vi "New Project.vi"(9 "DBSet":T1={"Server"="172.20.23.107", "DB"="HTPSDB", "PSW"="data'songyy", "User"="sa"}, 10 "UserID":string="L043460", 11 "厂区":string="清溪") -> ()   [LabVIEW 2011] (continued)
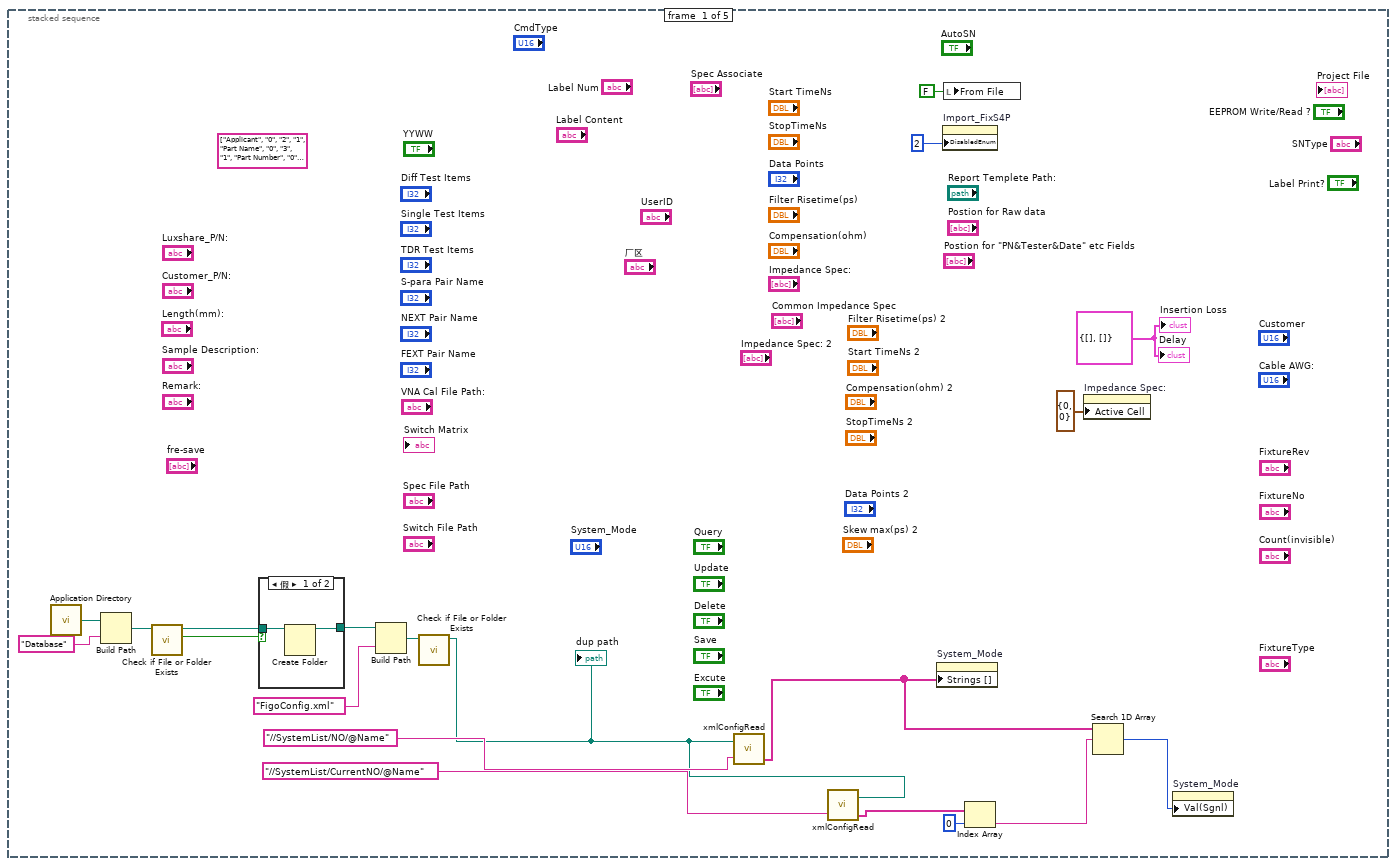
[diagram p3: hidden frame]
                            n930 = Build Array(w1122, w1135, w1134, w1133, w1132, w1131, w1130, w1129, w1128, w1127, w1110, w1112, w1123, w1126, w1138, w1125, w1124, w1119, w1107, w1108, w1109, w1105) -> (w1114:string[])
                            n931 = local write "Project File"(w1114) -> ()
                          }
                        }
                      }
                      frame #4 {
                        n932 = local read "save?"() -> (w1140:bool)
                        n933 = case shown="真" w1140 {
                          tunnel: w1139 -> [_ w1142]
                          frame False {
                            n934 = One Button Dialog(message="保存信息不完整" ("消息")) -> ()  [unwired: 1 in, 1 out]
                          }
                          frame True {
                            n935 = local read "Luxshare_P/N:"() -> (w1145:string)
                            n936 = local read "Project File"() -> (w1144:string[])
                            n937 = local read "Local"() -> (w1143:bool)
                            n938 = case shown="真" w1143 {
                              tunnel: w1144 -> [w1150 w1162]
                              tunnel: w1145 -> [_ w1170]
                              tunnel: w1142 -> [w1146 _]
                              frame False {
                                (unwired) string[] ["LuxsharePN", "CustomerPN", "Customer", "Prjinf", "SampleDes", "AWG", "Length", "Spec", "SwitchMatrix", "EEPROMTF", "FixtureNo", "LabelTF", "LabelNum", "LabelC", "Remark", "AutoSN", "FrePoints"] ("列名")
                                # "保存至数据库"
                                n939 = call "sql-writeinfo_vproject.vi"("操作模式"=enum16{"写入数据", "更改数据"}."写入数据", "列名"=string[] ["LuxsharePN", "CustomerPN", "Customer", "Prjinf", "SampleDes", "AWG", "Length", "Spec", "SwitchMatrix", "EEPROMTF", "FixtureNo", "LabelTF", "LabelNum", "LabelC", "Remark", "AutoSN", "FrePoints", "Switch_File_Path", "Spec_File_Path", "Spec_Points", "HardWare_Mode", "Factory", "LastLog"], "DBSet"=w1146, "值"=w1150) -> ("简单报错"=w1148:string, "status"=w1149:bool)  [unwired: 14 in]
                                n940 = case shown="假" w1149 {
                                tunnel: w1148 -> [_ w1161]
                                frame False {
                                # "清空操作"
                                n941 = control-ref of="Spec Associate"() -> (w1152:refnum<vi>)
                                n942 = control-ref of="Report Templete Path:"() -> (w1155:refnum<vi>)
                                n943 = control-ref of="Data Points"() -> (w1154:refnum<vi>)
                                n944 = local read "bool"() -> (w1153:refnum<vi>[])
                                n945 = One Button Dialog(message="Save Finished!" ("消息")) -> ()  [unwired: 1 in, 1 out]
                                n946 = local read "number"() -> (w1156:refnum<vi>[])
                                n947 = local read "string"() -> (w1159:refnum<vi>[])
                                n948 = local read "chart"() -> (w1157:refnum<vi>[])
                                n949 = local read "list"() -> (w1158:refnum<vi>[])
                                n950 = call "_wmg_initAllCtrls.vi"("chart"=w1157, "number"=w1156, "list"=w1158, "string"=w1159, "bool"=w1153, "Spec _Data"=w1152, "Data Points"=w1154, "Report Templete Path:"=w1155) -> ()
                                }
                                frame True {
                                n951 = One Button Dialog(message=w1161) -> ()  [unwired: 1 in, 1 out]
                                }
                                }
                              }
                              frame True {
                                n952 = call <vilib>:"Application Directory.vi"() -> ("Application Directory"=w1169:path)
                                n953 = Concatenate Strings("Database\\" ("字符串"), w1170, ".hpj" ("字符串")) -> (w1168:string)
                                n954 = Build Path(base path=w1169, name or relative path=w1168) -> (appended path=w1165:path)
                                n955 = call <vilib>:"Check if File or Folder Exists.vi"("path"=w1165) -> ("file or folder exists?"=w1164:bool, "dup path"=w1163:path)  [unwired: 8 in, 1 out]
                                n956 = case shown="真" w1164 {
                                tunnel: w1163 -> [w1174 w1184]
                                tunnel: w1162 -> [w1173 w1183]
                                frame False {
                                # "清空操作"
                                n957 = control-ref of="Spec Associate"() -> (w1171:refnum<vi>)
                                n958 = One Button Dialog(message="Local file save Finished!" ("消息")) -> ()  [unwired: 1 in, 1 out]
                                n959 = control-ref of="Report Templete Path:"() -> (w1180:refnum<vi>)
                                n960 = control-ref of="Data Points"() -> (w1181:refnum<vi>)
                                n961 = local read "bool"() -> (w1172:refnum<vi>[])
                                n962 = Write to Binary File(file (use dialog)=w1174, data=w1173, 9:T8."big-endian, network order" ("字节顺序(0:big-endian, network order)")) -> ()  [unwired: 3 in, 3 out]
                                n963 = local read "number"() -> (w1179:refnum<vi>[])
                                n964 = local read "string"() -> (w1176:refnum<vi>[])
                                n965 = local read "chart"() -> (w1178:refnum<vi>[])
                                n966 = local read "list"() -> (w1177:refnum<vi>[])
                                n967 = call "_wmg_initAllCtrls.vi"("chart"=w1178, "number"=w1179, "list"=w1177, "string"=w1176, "bool"=w1172, "Spec _Data"=w1171, "Data Points"=w1181, "Report Templete Path:"=w1180) -> ()
                                }
                                frame True {
                                n968 = Two Button Dialog(message="该PN的文件已经存在\n是否覆盖？", 1:"取消" ("F按钮名称（“取消”）"), 2:"覆盖" ("T按钮名称（“确定”）")) -> (T button?=w1185:bool)
                                n969 = case shown="真" w1185 {
                                tunnel: w1184 -> [_ w1190]
                                tunnel: w1183 -> [_ w1189]
                                frame False {
                                }
                                frame True {
                                n970 = stacked-sequence {
                                tunnel: w1190 -> [w1193 _]
                                tunnel: w1189 -> [w1191 _]
                                frame #0 {
                                n971 = One Button Dialog(message="Coved successfully!" ("消息")) -> ()  [unwired: 1 in, 1 out]
                                n972 = Write to Binary File(file (use dialog)=w1193, data=w1191, 9:T8."big-endian, network order" ("字节顺序(0:big-endian, network order)")) -> ()  [unwired: 3 in, 3 out]
                                }
                                frame #1 {
                                # "清空操作"
                                n973 = control-ref of="Report Templete Path:"() -> (w1200:refnum<vi>)
                                n974 = control-ref of="Data Points"() -> (w1201:refnum<vi>)
                                n975 = control-ref of="Spec Associate"() -> (w1195:refnum<vi>)
                                n976 = local read "number"() -> (w1199:refnum<vi>[])
                                n977 = local read "string"() -> (w1196:refnum<vi>[])
                                n978 = local read "chart"() -> (w1198:refnum<vi>[])
                                n979 = local read "list"() -> (w1197:refnum<vi>[])
                                n980 = call "_wmg_initAllCtrls.vi"("chart"=w1198, "number"=w1199, "list"=w1197, "string"=w1196, "Spec _Data"=w1195, "Data Points"=w1201, "Report Templete Path:"=w1200) -> ()  [unwired: 1 in]
                                }
                                }
                                }
                                }
                                }
                                }
                              }
                            }
                          }
                        }
                      }
                      frame #5 {
                        n981 = property on="Update" class="Bool (严格)"("DisabledEnum"=T5."Disabled and Grayed Out" ("禁用")) -> ()  [unwired: 2 in, 2 out]
                        n982 = property on="Delete" class="Bool (严格)"("DisabledEnum"=T5."Disabled and Grayed Out" ("禁用")) -> ()  [unwired: 2 in, 2 out]
                        n983 = property on="Luxshare_P/N:" class="Str"("DisabledEnum"=T5."Disabled and Grayed Out" ("禁用")) -> ()  [unwired: 2 in, 2 out]
                        n984 = local write "Delete"(FALSE ("Query")) -> ()
                        n985 = local write "Save"(FALSE ("Query")) -> ()
                        n986 = local write "Query"(FALSE ("Query")) -> ()
                        n987 = local write "Update"(FALSE ("Query")) -> ()
                      }
                    }
                  }
                  frame #2 {
                    w1210 = u16 0 items=["", "Common", "H3C psw 10G", "H3C psw 28G"] ("CmdType")
                    # "清空数组"
                    n988 = control-ref of="Spec Associate"() -> (w1209:refnum<vi>)
                    n989 = control-ref of="Report Templete Path:"() -> (w1213:refnum<vi>)
                    n990 = control-ref of="Data Points"() -> (w1212:refnum<vi>)
                    n991 = local write "CmdType"(w1210) -> ()
                    n992 = local read "bool"() -> (w1211:refnum<vi>[])
                    n993 = local read "number"() -> (w1214:refnum<vi>[])
                    n994 = local read "string"() -> (w1217:refnum<vi>[])
                    n995 = local read "chart"() -> (w1215:refnum<vi>[])
                    n996 = local read "list"() -> (w1216:refnum<vi>[])
                    n997 = call "_wmg_initAllCtrls.vi"("chart"=w1215, "number"=w1214, "list"=w1216, "string"=w1217, "bool"=w1211, "Spec _Data"=w1209, "Data Points"=w1212, "Report Templete Path:"=w1213) -> ()
                    n998 = property on="Update" class="Bool (严格)"("DisabledEnum"=T5."Disabled and Grayed Out" ("禁用")) -> ()  [unwired: 2 in, 2 out]
                    n999 = property on="Delete" class="Bool (严格)"("DisabledEnum"=T5."Disabled and Grayed Out" ("禁用")) -> ()  [unwired: 2 in, 2 out]
                    n1000 = property on="Luxshare_P/N:" class="Str"("DisabledEnum"=T5."Disabled and Grayed Out" ("禁用")) -> ()  [unwired: 2 in, 2 out]
                    n1001 = local write "Delete"(FALSE ("Query")) -> ()
                    n1002 = local write "Save"(FALSE ("Query")) -> ()
                    n1003 = local write "Query"(FALSE ("Query")) -> ()
                    n1004 = local write "Update"(FALSE ("Query")) -> ()
                  }
                }
              }
              frame 10 {
                n1005 = stacked-sequence {
                  tunnel: w1225 -> [w1226 _]
                  frame #0 {
                    n1006 = local read "Local"() -> (w1227:bool)
                    n1007 = case shown="假" w1227 {
                      tunnel: w1226 -> [w1228 _]
                      frame False {
                        n1008 = local read "Luxshare_P/N:"() -> (w1237:string)
                        n1009 = property on="System_Mode" class="Ring (严格)"() -> ("RingText.Text"=w1233:string)  [unwired: 2 in, 2 out]
                        n1010 = local read "厂区"() -> (w1229:string)
                        n1011 = call "_wmg_HardModetoHardModewhereConnect.vi"("Input"=w1233, "Factory"=w1229) -> ("Output"=w1231:string)
                        n1012 = call "_wmg_PNtoPNwhereConnect.vi"("Input"=w1237) -> ("Output"=w1232:string)
                        n1013 = Concatenate Strings(w1232, w1231) -> (w1230:string)
                        n1014 = call "sql-delete.vi"("操作模式"=T9."删除数据", "DBSet"=w1228, "限定条件"=w1230) -> ("错误类型"=w1234:string, "status"=w1235:bool)  [unwired: 15 in]
                        n1015 = case shown="假" w1235 {
                          tunnel: ["数据删除成功！" ("消息") w1240] -> w1236
                          tunnel: w1234 -> [_ w1240]
                          frame False {
                          }
                          frame True {
                          }
                        }
                        n1016 = One Button Dialog(message=w1236) -> ()  [unwired: 1 in, 1 out]
                      }
                      frame True {
                        n1017 = local read "Luxshare_P/N:"() -> (w1246:string)
                        n1018 = call <vilib>:"Application Directory.vi"() -> ("Application Directory"=w1250:path)
                        n1019 = Concatenate Strings("Database\\" ("字符串"), w1246, ".hpj" ("字符串")) -> (w1249:string)
                        n1020 = Build Path(base path=w1250, name or relative path=w1249) -> (appended path=w1245:path)
                        n1021 = Delete(path (use dialog)=w1245) -> (error out=w1241:errorcluster)  [unwired: 4 in, 2 out]
                        n1022 = Unbundle(w1241) -> ("status"=w1244:bool, "source"=w1242:string)  [unwired: 1 out]
                        n1023 = case shown="假" w1244 {
                          tunnel: ["文件删除成功！" ("消息") w1252] -> w1243
                          tunnel: w1242 -> [_ w1252]
                          frame False {
                          }
                          frame True {
                          }
                        }
                        n1024 = One Button Dialog(message=w1243) -> ()  [unwired: 1 in, 1 out]
                      }
                    }
                  }
                  frame #1 {
                    w1254 = u16 0 items=["", "Common", "H3C psw 10G", "H3C psw 28G"] ("CmdType")
                    # "清空数组"
                    n1025 = control-ref of="Spec Associate"() -> (w1253:refnum<vi>)
                    n1026 = control-ref of="Report Templete Path:"() -> (w1264:refnum<vi>)
                    n1027 = control-ref of="Data Points"() -> (w1263:refnum<vi>)
                    n1028 = local write "CmdType"(w1254) -> ()
                    n1029 = local read "bool"() -> (w1255:refnum<vi>[])
                    n1030 = local read "number"() -> (w1265:refnum<vi>[])
                    n1031 = local read "string"() -> (w1268:refnum<vi>[])
                    n1032 = local read "chart"() -> (w1266:refnum<vi>[])
                    n1033 = local read "list"() -> (w1267:refnum<vi>[])
                    n1034 = call "_wmg_initAllCtrls.vi"("chart"=w1266, "number"=w1265, "list"=w1267, "string"=w1268, "bool"=w1255, "Spec _Data"=w1253, "Data Points"=w1263, "Report Templete Path:"=w1264) -> ()
                    n1035 = local write "Delete"(FALSE ("Query")) -> ()
                    n1036 = property on="Update" class="Bool (严格)"("DisabledEnum"=T5."Disabled and Grayed Out" ("禁用")) -> ()  [unwired: 2 in, 2 out]
                    n1037 = property on="Delete" class="Bool (严格)"("DisabledEnum"=T5."Disabled and Grayed Out" ("禁用")) -> ()  [unwired: 2 in, 2 out]
                    n1038 = property on="Luxshare_P/N:" class="Str"("DisabledEnum"=T5."Disabled and Grayed Out" ("禁用")) -> ()  [unwired: 2 in, 2 out]
                    n1039 = local write "Save"(FALSE ("Query")) -> ()
                    n1040 = local write "Query"(FALSE ("Query")) -> ()
                    n1041 = local write "Update"(FALSE ("Query")) -> ()
                  }
                }
              }
              frame 1 {
                n1042 = stacked-sequence {
                  tunnel: w1269 -> [_ _ _ _ w1451 _]
                  frame #0 {
                    w1296 = "@"
                    w1297 = "\r\n"
                    w1307 = "%s" ("格式字符串")
                    n1043 = local read "Impedance Spec:"() -> (w1309:string[][])
                    n1044 = local read "2X Thru String"() -> (w1293:string)
                    n1045 = property on="Delay(ns)" class="DigNum (严格)"() -> ("NumText.Text"=w1291:string)  [unwired: 2 in, 2 out]
                    n1046 = property on="Skew max(ps)" class="DigNum (严格)"() -> ("NumText.Text"=w1292:string)  [unwired: 2 in, 2 out]
                    n1047 = Boolean To (0,1)(Boolean="Impedance Filter") -> (0, 1=w1312:i16)
                    n1048 = property on="Filter Risetime(ps)" class="DigNum (严格)"() -> ("NumText.Text"=w1287:string)  [unwired: 2 in, 2 out]
                    n1049 = property on="Start TimeNs" class="DigNum (严格)"() -> ("NumText.Text"=w1290:string)  [unwired: 2 in, 2 out]
                    n1050 = property on="StopTimeNs" class="DigNum (严格)"() -> ("NumText.Text"=w1289:string)  [unwired: 2 in, 2 out]
                    n1051 = property on="Data Points" class="DigNum (严格)"() -> ("NumText.Text"=w1288:string)  [unwired: 2 in, 2 out]
                    n1052 = property on="Compensation(ohm)" class="DigNum (严格)"() -> ("NumText.Text"=w1286:string)  [unwired: 2 in, 2 out]
                    n1053 = Number To Decimal String(number=w1312) -> (decimal integer string=w1310:string)  [unwired: 1 in]
                    n1054 = call "impedance spec.vi"("Impedance Spec:"=w1309) -> ("Impedance spec string"=w1308:string)  [unwired: 10 in]
                    n1055 = call <vilib>:"Trim Whitespace.vi"("string"=w1293) -> ("trimmed string"=w1285:string)  [unwired: 1 in]
                    n1056 = Build Array(w1290, w1289, w1288, w1287, w1286, w1310, w1308, w1291, w1292, w1285) -> (→"TDR Setting":string[])
                    n1057 = local read "Impedance Spec: 2"() -> (w1275:string[][])
                    n1058 = local read "Report Templete Path:"() -> (w1294:path)
                    n1059 = local read "2X Thru String"() -> (w1282:string)
                    n1060 = property on="Delay(ns)" class="DigNum (严格)"() -> ("NumText.Text"=w1273:string)  [unwired: 2 in, 2 out]
                    n1061 = property on="Skew max(ps) 2" class="DigNum (严格)"() -> ("NumText.Text"=w1272:string)  [unwired: 2 in, 2 out]
                    n1062 = property on="Postion for Raw data" class="Tbl (严格)"() -> ("Value"=w1306:string[][])  [unwired: 2 in, 2 out]
                    n1063 = property on="Start TimeNs 2" class="DigNum (严格)"() -> ("NumText.Text"=w1281:string)  [unwired: 2 in, 2 out]
                    n1064 = property on="StopTimeNs 2" class="DigNum (严格)"() -> ("NumText.Text"=w1280:string)  [unwired: 2 in, 2 out]
                    n1065 = property on="Data Points 2" class="DigNum (严格)"() -> ("NumText.Text"=w1279:string)  [unwired: 2 in, 2 out]
                    n1066 = property on="Postion for \"PN&Tester&Date\" etc Fields" class="Tbl (严格)"() -> ("Value"=w1305:string[][])  [unwired: 2 in, 2 out]
                    n1067 = property on="Filter Risetime(ps) 2" class="DigNum (严格)"() -> ("NumText.Text"=w1278:string)  [unwired: 2 in, 2 out]
                    n1068 = property on="Compensation(ohm) 2" class="DigNum (严格)"() -> ("NumText.Text"=w1277:string)  [unwired: 2 in, 2 out]
                    n1069 = Boolean To (0,1)(Boolean="Impedance Filter 2") -> (0, 1=w1283:i16)
                    n1070 = Array To Spreadsheet String(array=w1306, 3:w1307) -> (spreadsheet string=w1302:string)  [unwired: 1 in]
                    n1071 = Array To Spreadsheet String(array=w1305, 3:w1307) -> (spreadsheet string=w1300:string)  [unwired: 1 in]
                    n1072 = Number To Decimal String(number=w1283) -> (decimal integer string=w1276:string)  [unwired: 1 in]
                    n1073 = call "impedance spec.vi"("Impedance Spec:"=w1275) -> ("Impedance spec string"=w1274:string)  [unwired: 10 in]
                    n1074 = call <vilib>:"Trim Whitespace.vi"("string"=w1282) -> ("trimmed string"=w1271:string)  [unwired: 1 in]
                    n1075 = Path To String(path=w1294) -> (string=w1295:string)
                    n1076 = Search and Replace String(replace all?=TRUE ("替换全部？(F)"), input string=w1302, search string=w1297, replace string=w1296) -> (result string=w1299:string)  [unwired: 4 in, 3 out]
                    n1077 = Search and Replace String(replace all?=TRUE ("替换全部？(F)"), input string=w1300, search string=w1297, replace string=w1296) -> (result string=w1298:string)  [unwired: 4 in, 3 out]
                    n1078 = Build Array(w1281, w1280, w1279, w1278, w1277, w1276, w1274, w1273, w1272, w1271) -> (→"TDR Setting2":string[])
                    n1079 = Build Array(w1295, w1299, w1298) -> (→"Report Config":string[])
                  }
                  frame #1 {
                    n1080 = property on="S-para Pair Name" class="LstBox (严格)"() -> ("Item Names"=w1349:string[], "Item Symbols"=w1348:i32[])  [unwired: 2 in, 2 out]
                    n1081 = property on="NEXT Pair Name" class="LstBox (严格)"() -> ("Item Names"=w1347:string[], "Item Symbols"=w1346:i32[])  [unwired: 2 in, 2 out]
                    n1082 = local read "Common Impedance Spec"() -> (w1317:string[][])
                    n1083 = property on="FEXT Pair Name" class="LstBox (严格)"() -> ("Item Names"=w1345:string[], "Item Symbols"=w1344:i32[])  [unwired: 2 in, 2 out]
                    n1084 = property on="Single Test Items" class="LstBox (严格)"() -> ("Item Names"=w1351:string[], "Item Symbols"=w1350:i32[])  [unwired: 2 in, 2 out]
                    n1085 = property on="Diff Test Items" class="LstBox (严格)"() -> ("Item Names"=w1353:string[], "Item Symbols"=w1352:i32[])  [unwired: 2 in, 2 out]
                    n1086 = property on="TDR Test Items" class="LstBox (严格)"() -> ("Item Names"=w1329:string[], "Item Symbols"=w1328:i32[])  [unwired: 2 in, 2 out]
                    n1087 = call "Selected items.vi"("Item Syms"=w1348, "Item name"=w1349) -> ("Selected tem"=w1343:string[])  [unwired: 7 in, 2 out]
                    n1088 = call "Selected items.vi"("Item Syms"=w1346, "Item name"=w1347) -> ("Selected tem"=w1342:string[])  [unwired: 7 in, 2 out]
                    n1089 = call "Selected items.vi"("Item Syms"=w1344, "Item name"=w1345) -> ("Selected tem"=w1341:string[])  [unwired: 7 in, 2 out]
                    n1090 = call "Selected items.vi"("Item Syms"=w1352, "Item name"=w1353) -> ("Selected tem"=w1340:string[])  [unwired: 7 in, 2 out]
                    n1091 = call "Selected items.vi"("Item Syms"=w1350, "Item name"=w1351) -> ("Selected tem"=w1339:string[])  [unwired: 7 in, 2 out]
                    n1092 = call "Selected items.vi"("Item Syms"=w1328, "Item name"=w1329) -> ("Selected tem"=w1327:string[])  [unwired: 7 in, 2 out]
                    n1093 = call "impedance spec.vi"("Impedance Spec:"=w1317) -> ("Impedance spec string"=w1316:string)  [unwired: 10 in]
                    n1094 = local read "VNA Cal File Path:"() -> (w1324:string)
                    n1095 = Build Array(w1316) -> (w1315:string[])
                    n1096 = local read "Report Config"() -> (w1325:string[])
                    n1097 = local read "Cancel Dem2X?"() -> (w1322:bool)
                    n1098 = local read "TDR Setting2"() -> (w1323:string[])
                    n1099 = local read "TDR Setting"() -> (w1326:string[])
                    n1100 = Build Array(w1324) -> (w1338:string[])
                    n1101 = Number To Decimal String(number="ILD Spec") -> (decimal integer string=w1331:string)  [unwired: 1 in]
                    n1102 = Build Array(w1331) -> (w1330:string[])
                    n1103 = Select(t="TRUE", s=w1322, f="FALSE") -> (s? t:f=w1319:string)
                    n1104 = Build Array(w1319) -> (w1318:string[])
                    n1105 = Build Array(w1343, w1342, w1341, w1340, w1339, w1327, string[] ["占位符"], w1338, w1325, w1330, w1326, w1323, w1318, w1315) -> (w1337:string[][])
                    n1106 = Transpose 2D Array(2D array=w1337) -> (transposed array=w1336:string[][])
                    n1107 = Array To Spreadsheet String(delimiter (Tab)="#" ("分隔符(Tab)"), array=w1336, 3:"%s" ("格式字符串")) -> (spreadsheet string=→"Project Information":string)
                  }
                  frame #2 {
                    n1108 = local read "VNA Cal File Path:"() -> (w1373:string)
                    n1109 = property on="Diff Test Items" class="LstBox (严格)"() -> ("Item Symbols"=w1370:i32[])  [unwired: 2 in, 2 out]
                    n1110 = property on="Single Test Items" class="LstBox (严格)"() -> ("Item Symbols"=w1369:i32[])  [unwired: 2 in, 2 out]
                    n1111 = property on="TDR Test Items" class="LstBox (严格)"() -> ("Item Symbols"=w1368:i32[])  [unwired: 2 in, 2 out]
                    n1112 = property on="S-para Pair Name" class="LstBox (严格)"() -> ("Item Symbols"=w1367:i32[])  [unwired: 2 in, 2 out]
                    n1113 = property on="NEXT Pair Name" class="LstBox (严格)"() -> ("Item Symbols"=w1366:i32[])  [unwired: 2 in, 2 out]
                    n1114 = property on="FEXT Pair Name" class="LstBox (严格)"() -> ("Item Symbols"=w1362:i32[])  [unwired: 2 in, 2 out]
                    n1115 = local read "Luxshare_P/N:"() -> (w1360:string)
                    n1116 = local read "Length(mm):"() -> (w1374:string)
                    n1117 = String Length(string=w1360) -> (length=w1361:i32)
                    n1118 = Empty String/Path?(string/path=w1373) -> (empty?=w1371:bool)
                    n1119 = Empty String/Path?(string/path=w1374) -> (empty?=w1372:bool)
                    n1120 = Build Array(w1370, w1369, w1368, w1367, w1366, w1362) -> (w1365:i32[][])
                    n1121 = Not(x=w1372) -> (.not. x?=w1364:bool)
                    n1122 = Not(x=w1371) -> (.not. x?=w1363:bool)
                    n1123 = Greater Than 0?(x=w1361) -> (x > 0?=w1359:bool)
                    n1124 = local read "Spec Associate"() -> (w1354:string[][])
                    n1125 = call "_wmg_whetherItemsEmpty.vi"("Input"=w1365) -> ("bool"=w1375:bool)
                    n1126 = Compound Arithmetic op=AND(w1359, w1364, w1363, w1375) -> (→"save?":bool)
                    n1127 = Array To Spreadsheet String(delimiter (Tab)="#" ("分隔符(Tab)"), array=w1354, 3:"%s" ("格式字符串")) -> (spreadsheet string=w1357:string)
                    n1128 = local write "Spec String"(w1357) -> ()
                  }
                  frame #3 {
                    n1129 = local read "Local"() -> (w1376:bool)
                    n1130 = case shown="真" w1376 {
                      frame False {
                        # "16"
                        # "15"
                        # "14"
                        # "13"
                        # "11"
                        # "10"
                        # "9"
                        # "8"
                        # "7"
                        # "6"
                        # "5"
                        # "4"
                        # "3"
                        # "2"
                        # "1"
                        n1131 = local read "Label Print?"() -> (w1388:bool)
                        n1132 = local read "UserID"() -> (w1380:string)
                        n1133 = local read "fre-save"() -> (w1395:string[])
                        n1134 = Format Date/Time String(time format string (%c)="%Y-%m-%d : %H:%M" ("时间格式字符串(%c)")) -> (date/time string=w1377:string)  [unwired: 2 in]
                        n1135 = Boolean To (0,1)(Boolean=w1388) -> (0, 1=w1413:i16)
                        n1136 = local read "EEPROM Write/Read ?"() -> (w1389:bool)
                        n1137 = local read "Sample Description:"() -> (w1409:string)
                        n1138 = local read "Project Information"() -> (w1410:string)
                        n1139 = Array To Spreadsheet String(delimiter (Tab)="," ("分隔符(Tab)"), array=w1395, 3:"" ("格式字符串")) -> (spreadsheet string=w1392:string)
                        n1140 = Number To Decimal String(number=w1413) -> (decimal integer string=w1403:string)  [unwired: 1 in]
                        n1141 = local read "Customer_P/N:"() -> (w1412:string)
                        n1142 = local read "Switch Matrix"() -> (w1405:string)
                        n1143 = local read "Label Content"() -> (w1402:string)
                        n1144 = local read "Length(mm):"() -> (w1407:string)
                        n1145 = local read "Spec String"() -> (w1406:string)
                        n1146 = call <vilib>:"Trim Whitespace.vi"("string"=w1392) -> ("trimmed string"=w1391:string)  [unwired: 1 in]
                        n1147 = Concatenate Strings(w1380, " saved@" ("字符串"), w1377) -> (w1379:string)
                        n1148 = property on="Customer" class="Ring (严格)"() -> ("RingText.Text"=w1411:string)  [unwired: 2 in, 2 out]
                        n1149 = property on="Cable AWG:" class="Ring (严格)"() -> ("RingText.Text"=w1408:string)  [unwired: 2 in, 2 out]
                        n1150 = local read "FixtureNo"() -> (w1400:string)
                        n1151 = local read "Label Num"() -> (w1415:string)
                        n1152 = local read "Remark:"() -> (w1401:string)
                        n1153 = local read "厂区"() -> (w1382:string)
                        n1154 = local read "Switch File Path"() -> (w1387:string)
                        n1155 = Boolean To (0,1)(Boolean=w1389) -> (0, 1=w1414:i16)
                        n1156 = local read "AutoSN"() -> (w1397:bool)
                        n1157 = Number To Decimal String(number=w1414) -> (decimal integer string=w1404:string)  [unwired: 1 in]
                        n1158 = Boolean To (0,1)(Boolean=w1397) -> (0, 1=w1398:i16)
                        n1159 = local read "Spec File Path"() -> (w1386:string)
                        n1160 = Number To Decimal String(number=w1398) -> (decimal integer string=w1396:string)  [unwired: 1 in]
                        n1161 = local read "Luxshare_P/N:"() -> (w1399:string)
                        n1162 = local read "Spec Points"() -> (w1385:dbl)
                        n1163 = property on="System_Mode" class="Ring (严格)"() -> ("RingText.Text"=w1383:string)  [unwired: 2 in, 2 out]
                        n1164 = Number To Decimal String(number=w1385) -> (decimal integer string=w1384:string)  [unwired: 1 in]
                        n1165 = Build Array(w1399, w1412, w1411, w1410, w1409, w1408, w1407, w1406, w1405, w1404, w1400, w1403, w1415, w1402, w1401, w1396, w1391, w1387, w1386, w1384, w1383, w1382, w1379) -> (w1390:string[])
                        n1166 = local write "Project File"(w1390) -> ()
                      }
                      frame True {
                        # "11"
                        # "10"
                        # "9"
                        # "8"
                        # "7"
                        # "6"
                        # "5"
                        # "4"
                        # "3"
                        # "2"
                        # "1"
                        n1167 = local read "Label Print?"() -> (w1421:bool)
                        n1168 = local read "fre-save"() -> (w1429:string[])
                        n1169 = Boolean To (0,1)(Boolean=w1421) -> (0, 1=w1448:i16)
                        n1170 = local read "EEPROM Write/Read ?"() -> (w1423:bool)
                        n1171 = property on="CmdType" class="Ring (严格)"() -> ("RingText.Text"=w1420:string)  [unwired: 2 in, 2 out]
                        n1172 = local read "Sample Description:"() -> (w1444:string)
                        n1173 = local read "Project Information"() -> (w1445:string)
                        n1174 = Array To Spreadsheet String(delimiter (Tab)="," ("分隔符(Tab)"), array=w1429, 3:"" ("格式字符串")) -> (spreadsheet string=w1426:string)
                        n1175 = local read "SNType"() -> (w1422:string)
                        n1176 = Number To Decimal String(number=w1448) -> (decimal integer string=w1438:string)  [unwired: 1 in]
                        n1177 = local read "Customer_P/N:"() -> (w1447:string)
                        n1178 = local read "Switch Matrix"() -> (w1440:string)
                        n1179 = local read "Label Content"() -> (w1437:string)
                        n1180 = local read "Length(mm):"() -> (w1442:string)
                        n1181 = local read "Spec String"() -> (w1441:string)
                        n1182 = call <vilib>:"Trim Whitespace.vi"("string"=w1426) -> ("trimmed string"=w1425:string)  [unwired: 1 in]
                        n1183 = property on="Customer" class="Ring (严格)"() -> ("RingText.Text"=w1446:string)  [unwired: 2 in, 2 out]
                        n1184 = property on="Cable AWG:" class="Ring (严格)"() -> ("RingText.Text"=w1443:string)  [unwired: 2 in, 2 out]
                        n1185 = local read "FixtureNo"() -> (w1435:string)
                        n1186 = local read "Label Num"() -> (w1450:string)
                        n1187 = local read "Remark:"() -> (w1436:string)
                        n1188 = call <vilib>:"Trim Whitespace.vi"("string"=w1420) -> ("trimmed string"=w1433:string)  [unwired: 1 in]
                        n1189 = local read "Switch File Path"() -> (w1419:string)
                        n1190 = Boolean To (0,1)(Boolean=w1423) -> (0, 1=w1449:i16)
                        n1191 = local read "AutoSN"() -> (w1431:bool)
                        n1192 = Number To Decimal String(number=w1449) -> (decimal integer string=w1439:string)  [unwired: 1 in]
                        n1193 = Boolean To (0,1)(Boolean=w1431) -> (0, 1=w1432:i16)
                        n1194 = Number To Decimal String(number=w1432) -> (decimal integer string=w1430:string)  [unwired: 1 in]
                        n1195 = local read "Luxshare_P/N:"() -> (w1434:string)
                        n1196 = local read "Spec File Path"() -> (w1418:string)
                        n1197 = local read "Spec Points"() -> (w1417:dbl)
                        n1198 = Number To Decimal String(number=w1417) -> (decimal integer string=w1416:string)  [unwired: 1 in]
                        n1199 = Build Array(w1434, w1447, w1446, w1445, w1444, w1443, w1442, w1441, w1440, w1439, w1433, w1422, w1435, w1438, w1450, w1437, w1436, w1430, w1425, w1419, w1418, w1416) -> (w1424:string[])
                        n1200 = local write "Project File"(w1424) -> ()
                      }
                    }
                  }
                  frame #4 {
                    n1201 = local read "save?"() -> (w1452:bool)
                    n1202 = case shown="真" w1452 {
                      tunnel: w1451 -> [_ w1454]
                      frame False {
                        n1203 = One Button Dialog(message="保存信息不完整" ("消息")) -> ()  [unwired: 1 in, 1 out]
                      }
                      frame True {
                        n1204 = local read "Luxshare_P/N:"() -> (w1456:string)
                        n1205 = local read "Project File"() -> (w1455:string[])
                        n1206 = case shown="真" "Local" {
                          tunnel: w1455 -> [w1462 w1474]
                          tunnel: w1456 -> [_ w1482]
                          tunnel: w1454 -> [w1458 _]
                          frame False {
                            # "保存至数据库"
                            n1207 = call "sql-writeinfo_vproject.vi"("操作模式"=enum16{"写入数据", "更改数据"}."写入数据", "列名"=string[] ["LuxsharePN", "CustomerPN", "Customer", "Prjinf", "SampleDes", "AWG", "Length", "Spec", "SwitchMatrix", "EEPROMTF", "FixtureNo", "LabelTF", "LabelNum", "LabelC", "Remark", "AutoSN", "FrePoints", "Switch_File_Path", "Spec_File_Path", "Spec_Points", "HardWare_Mode", "Factory", "LastLog"], "DBSet"=w1458, "值"=w1462) -> ("简单报错"=w1460:string, "status"=w1461:bool)  [unwired: 14 in]
                            n1208 = case shown="假" w1461 {
                              tunnel: w1460 -> [_ w1473]
                              frame False {
                                # "清空操作"
                                n1209 = control-ref of="Spec Associate"() -> (w1464:refnum<vi>)
                                n1210 = control-ref of="Report Templete Path:"() -> (w1467:refnum<vi>)
                                n1211 = control-ref of="Data Points"() -> (w1466:refnum<vi>)
                                n1212 = local read "bool"() -> (w1465:refnum<vi>[])
                                n1213 = One Button Dialog(message="Save Finished!" ("消息")) -> ()  [unwired: 1 in, 1 out]
                                n1214 = local read "number"() -> (w1468:refnum<vi>[])
                                n1215 = local read "string"() -> (w1471:refnum<vi>[])
                                n1216 = local read "chart"() -> (w1469:refnum<vi>[])
                                n1217 = local read "list"() -> (w1470:refnum<vi>[])
                                n1218 = call "_wmg_initAllCtrls.vi"("chart"=w1469, "number"=w1468, "list"=w1470, "string"=w1471, "bool"=w1465, "Spec _Data"=w1464, "Data Points"=w1466, "Report Templete Path:"=w1467) -> ()
                              }
                              frame True {
                                n1219 = One Button Dialog(message=w1473) -> ()  [unwired: 1 in, 1 out]
                              }
                            }
                          }
                          frame True {
                            n1220 = call <vilib>:"Application Directory.vi"() -> ("Application Directory"=w1481:path)
                            n1221 = Concatenate Strings("Database\\" ("字符串"), w1482, ".hpj" ("字符串")) -> (w1480:string)
                            n1222 = Build Path(base path=w1481, name or relative path=w1480) -> (appended path=w1477:path)
                            n1223 = call <vilib>:"Check if File or Folder Exists.vi"("path"=w1477) -> ("file or folder exists?"=w1476:bool, "dup path"=w1475:path)  [unwired: 8 in, 1 out]
                            n1224 = case shown="假" w1476 {
                              tunnel: w1475 -> [w1486 w1496]
                              tunnel: w1474 -> [w1485 w1495]
                              frame False {
                                # "清空操作"
                                n1225 = control-ref of="Spec Associate"() -> (w1483:refnum<vi>)
                                n1226 = One Button Dialog(message="Local file save Finished!" ("消息")) -> ()  [unwired: 1 in, 1 out]
                                n1227 = control-ref of="Report Templete Path:"() -> (w1492:refnum<vi>)
                                n1228 = control-ref of="Data Points"() -> (w1493:refnum<vi>)
                                n1229 = local read "bool"() -> (w1484:refnum<vi>[])
                                n1230 = Write to Binary File(file (use dialog)=w1486, data=w1485, 9:T8."big-endian, network order" ("字节顺序(0:big-endian, network order)")) -> ()  [unwired: 3 in, 3 out]
                                n1231 = local read "number"() -> (w1491:refnum<vi>[])
                                n1232 = local read "string"() -> (w1488:refnum<vi>[])
                                n1233 = local read "chart"() -> (w1490:refnum<vi>[])
                                n1234 = local read "list"() -> (w1489:refnum<vi>[])
                                n1235 = call "_wmg_initAllCtrls.vi"("chart"=w1490, "number"=w1491, "list"=w1489, "string"=w1488, "bool"=w1484, "Spec _Data"=w1483, "Data Points"=w1493, "Report Templete Path:"=w1492) -> ()
                              }
                              frame True {
                                n1236 = Two Button Dialog(message="该PN的文件已经存在\n是否覆盖？", 1:"取消" ("F按钮名称（“取消”）"), 2:"覆盖" ("T按钮名称（“确定”）")) -> (T button?=w1497:bool)
                                n1237 = case shown="真" w1497 {
                                tunnel: w1496 -> [_ w1502]
                                tunnel: w1495 -> [_ w1501]
                                frame False {
                                }
                                frame True {
                                n1238 = stacked-sequence {
                                tunnel: w1502 -> [w1505 _]
                                tunnel: w1501 -> [w1503 _]
                                frame #0 {
                                n1239 = One Button Dialog(message="Coved successfully!" ("消息")) -> ()  [unwired: 1 in, 1 out]
                                n1240 = Write to Binary File(file (use dialog)=w1505, data=w1503, 9:T8."big-endian, network order" ("字节顺序(0:big-endian, network order)")) -> ()  [unwired: 3 in, 3 out]
                                }
                                frame #1 {
                                # "清空操作"
                                n1241 = control-ref of="Report Templete Path:"() -> (w1512:refnum<vi>)
                                n1242 = control-ref of="Data Points"() -> (w1513:refnum<vi>)
                                n1243 = control-ref of="Spec Associate"() -> (w1507:refnum<vi>)
                                n1244 = local read "number"() -> (w1511:refnum<vi>[])
                                n1245 = local read "string"() -> (w1508:refnum<vi>[])
                                n1246 = local read "chart"() -> (w1510:refnum<vi>[])
                                n1247 = local read "list"() -> (w1509:refnum<vi>[])
                                n1248 = call "_wmg_initAllCtrls.vi"("chart"=w1510, "number"=w1511, "list"=w1509, "string"=w1508, "Spec _Data"=w1507, "Data Points"=w1513, "Report Templete Path:"=w1512) -> ()  [unwired: 1 in]
                                }
                                }
                                }
                                }
                              }
                            }
                          }
                        }
                      }
                    }
                  }
                  frame #5 {
                    w1514 = u16 0 items=["", "Common", "H3C psw 10G", "H3C psw 28G"] ("CmdType")
                    n1249 = property on="Update" class="Bool (严格)"("DisabledEnum"=T5."Disabled and Grayed Out" ("禁用")) -> ()  [unwired: 2 in, 2 out]
                    n1250 = property on="Delete" class="Bool (严格)"("DisabledEnum"=T5."Disabled and Grayed Out" ("禁用")) -> ()  [unwired: 2 in, 2 out]
                    n1251 = property on="Luxshare_P/N:" class="Str"("DisabledEnum"=T5."Disabled and Grayed Out" ("禁用")) -> ()  [unwired: 2 in, 2 out]
                    n1252 = local write "CmdType"(w1514) -> ()
                    n1253 = local write "Delete"(FALSE ("Query")) -> ()
                    n1254 = local write "Save"(FALSE ("Query")) -> ()
                    n1255 = local write "Query"(FALSE ("Query")) -> ()
                    n1256 = local write "Update"(FALSE ("Query")) -> ()
                  }
                }
              }
            }
          }
          event "System_Mode": Value Change {
            w1526 = "@NameVar@" ("搜索字符串")
            n1257 = event-data() -> ("NewVal"=w1535:u16)  [unwired: 1 in, 4 out]
            n1258 = property on="System_Mode" class="Ring (严格)"() -> ("Strings []"=w1536:string[])  [unwired: 2 in, 2 out]
            n1259 = local read "dup path"() -> (w1529:path)
            n1260 = Index Array(array=w1536, index=w1535) -> (element=w1522:string)
            n1261 = Search and Replace String(input string="//SystemList/NO[@Name='@NameVar@']/@Switch" ("XPath expression"), search string=w1526, replace string=w1522) -> (result string=w1533:string)  [unwired: 5 in, 3 out]
            n1262 = call "xmlConfigRead.vi"("path to XML document"=w1529, "XPath expression"=w1533) -> ("OutParaArray"=w1532:string[])  [unwired: 2 out]
            n1263 = Index Array(array=w1532, index=0 ("索引")) -> (element=→"开关型号":string)
            n1264 = Search and Replace String(input string="//SystemList/NO[@Name='@NameVar@']/@Equipment" ("XPath expression"), search string=w1526, replace string=w1522) -> (result string=w1528:string)  [unwired: 5 in, 3 out]
            n1265 = call "xmlConfigRead.vi"("path to XML document"=w1529, "XPath expression"=w1528) -> ("OutParaArray"=w1525:string[])  [unwired: 2 out]
            n1266 = Index Array(array=w1525, index=0 ("索引")) -> (element=→"仪器型号":string)
          }
          event Panel Close {
            n1267 = event-data() -> ()  [unwired: 1 in, 3 out]
          }
          event "Default": Value Change {
            n1268 = event-data() -> ()  [unwired: 1 in, 5 out]
            n1269 = case shown="\"Default\", 默认" "Default" {
              frame "Default", Default {
                w1539 = 0 ("Diff Test Items")
                w1545 = 37
                n1270 = local read "Inf"() -> (w1564:string[][])
                n1271 = Index Array(array=w1564, index (col) #1=0 ("禁用的索引 (列)"), index (col) #2=1 ("索引 (列)"), index (col) #3=2 ("索引 (列)"), index (col) #4=3 ("索引 (列)"), index (col) #5=4 ("索引 (列)"), index (col) #6=5 ("索引 (列)")) -> (element #1=w1558:string[], element #2=w1557:string[], element #3=w1556:string[], element #4=w1555:string[], element #5=w1554:string[], element #6=w1548:string[])  [unwired: 6 in]
                n1272 = call "Delete empty element from array.vi"("Array In"=w1548) -> ("Array out"=w1540:string[])  [unwired: 26 in]
                n1273 = call "Delete empty element from array.vi"("Array In"=w1558) -> ("Array out"=w1549:string[])  [unwired: 26 in]
                n1274 = call "Delete empty element from array.vi"("Array In"=w1554) -> ("Array out"=w1541:string[])  [unwired: 26 in]
                n1275 = call "Delete empty element from array.vi"("Array In"=w1557) -> ("Array out"=w1550:string[])  [unwired: 26 in]
                n1276 = call "Delete empty element from array.vi"("Array In"=w1556) -> ("Array out"=w1543:string[])  [unwired: 26 in]
                n1277 = call "Delete empty element from array.vi"("Array In"=w1555) -> ("Array out"=w1542:string[])  [unwired: 26 in]
                n1278 = Array Size(array=w1549) -> (size(s)=w1571:i32)
                n1279 = Array Size(array=w1550) -> (size(s)=w1565:i32)
                n1280 = Array Size(array=w1543) -> (size(s)=w1544:i32)
                n1281 = Array Size(array=w1542) -> (size(s)=w1551:i32)
                n1282 = Array Size(array=w1541) -> (size(s)=w1568:i32)
                n1283 = Array Size(array=w1540) -> (size(s)=w1552:i32)
                n1284 = Initialize Array(w1545, w1571) -> (w1570:i32[])
                n1285 = Initialize Array(w1545, w1565) -> (w1566:i32[])
                n1286 = Initialize Array(w1545, w1551) -> (w1569:i32[])
                n1287 = Initialize Array(w1545, w1544) -> (w1546:i32[])
                n1288 = Initialize Array(w1545, w1568) -> (w1567:i32[])
                n1289 = Initialize Array(w1545, w1552) -> (w1553:i32[])
                n1290 = property on="Diff Test Items" class="LstBox (严格)"("Item Names"=w1549, "Item Symbols"=w1570) -> ()  [unwired: 2 in, 2 out]
                n1291 = property on="Single Test Items" class="LstBox (严格)"("Item Names"=w1550, "Item Symbols"=w1566) -> ()  [unwired: 2 in, 2 out]
                n1292 = property on="TDR Test Items" class="LstBox (严格)"("Item Names"=w1543, "Item Symbols"=w1546) -> ()  [unwired: 2 in, 2 out]
                n1293 = property on="S-para Pair Name" class="LstBox (严格)"("Item Names"=w1542, "Item Symbols"=w1569) -> ()  [unwired: 2 in, 2 out]
                n1294 = property on="NEXT Pair Name" class="LstBox (严格)"("Item Names"=w1541, "Item Symbols"=w1567) -> ()  [unwired: 2 in, 2 out]
                n1295 = property on="FEXT Pair Name" class="LstBox (严格)"("Item Names"=w1540, "Item Symbols"=w1553) -> ()  [unwired: 2 in, 2 out]
                n1296 = property on="Diff Test Items" class="LstBox (严格)"("Value"=w1539, "Top Row"=w1539) -> ()  [unwired: 2 in, 2 out]
                n1297 = property on="Single Test Items" class="LstBox (严格)"("Value"=w1539, "Top Row"=w1539) -> ()  [unwired: 2 in, 2 out]
                n1298 = property on="TDR Test Items" class="LstBox (严格)"("Value"=w1539, "Top Row"=w1539) -> ()  [unwired: 2 in, 2 out]
                n1299 = property on="S-para Pair Name" class="LstBox (严格)"("Value"=w1539, "Top Row"=w1539) -> ()  [unwired: 2 in, 2 out]
                n1300 = property on="NEXT Pair Name" class="LstBox (严格)"("Value"=w1539, "Top Row"=w1539) -> ()  [unwired: 2 in, 2 out]
                n1301 = property on="FEXT Pair Name" class="LstBox (严格)"("Value"=w1539, "Top Row"=w1539) -> ()  [unwired: 2 in, 2 out]
              }
              frame "Quick" {
                w1572 = 0 ("Diff Test Items")
                w1576 = 38
                n1302 = local read "Inf"() -> (w1594:string[][])
                n1303 = Index Array(array=w1594, index (col) #1=0 ("禁用的索引 (列)"), index (col) #2=1 ("索引 (列)"), index (col) #3=3 ("索引 (列)"), index (col) #4=4 ("索引 (列)"), index (col) #5=5 ("索引 (列)")) -> (element #1=w1588:string[], element #2=w1587:string[], element #3=w1586:string[], element #4=w1585:string[], element #5=w1584:string[])  [unwired: 5 in]
                n1304 = call "Delete empty element from array.vi"("Array In"=w1588) -> ("Array out"=w1577:string[])  [unwired: 26 in]
                n1305 = call "Delete empty element from array.vi"("Array In"=w1584) -> ("Array out"=w1581:string[])  [unwired: 26 in]
                n1306 = call "Delete empty element from array.vi"("Array In"=w1587) -> ("Array out"=w1578:string[])  [unwired: 26 in]
                n1307 = call "Delete empty element from array.vi"("Array In"=w1586) -> ("Array out"=w1579:string[])  [unwired: 26 in]
                n1308 = call "Delete empty element from array.vi"("Array In"=w1585) -> ("Array out"=w1580:string[])  [unwired: 26 in]
                n1309 = Array Size(array=w1578) -> (size(s)=w1595:i32)
                n1310 = Array Size(array=w1580) -> (size(s)=w1598:i32)
                n1311 = Array Size(array=w1581) -> (size(s)=w1582:i32)
                n1312 = Initialize Array(37, w1595) -> (w1596:i32[])
                n1313 = Initialize Array(w1576, w1598) -> (w1597:i32[])
                n1314 = Initialize Array(w1576, w1582) -> (w1583:i32[])
                n1315 = property on="Diff Test Items" class="LstBox (严格)"("Item Names"=w1577, "Item Symbols"=i32[] [38, 37, 37, 38, 38, 37, 38, 37, 37, 37, 37, 37, 37, 37, 37, 37, 37, 37, 38, 38] ("初始化的数组")) -> ()  [unwired: 2 in, 2 out]
                n1316 = property on="Single Test Items" class="LstBox (严格)"("Item Names"=w1578, "Item Symbols"=w1596) -> ()  [unwired: 2 in, 2 out]
                n1317 = property on="S-para Pair Name" class="LstBox (严格)"("Item Names"=w1579, "Item Symbols"=i32[] [38, 38, 38, 38, 38, 38, 38, 38, 37, 37, 37, 37, 37, 37, 37, 37] ("初始化的数组")) -> ()  [unwired: 2 in, 2 out]
                n1318 = property on="NEXT Pair Name" class="LstBox (严格)"("Item Names"=w1580, "Item Symbols"=w1597) -> ()  [unwired: 2 in, 2 out]
                n1319 = property on="FEXT Pair Name" class="LstBox (严格)"("Item Names"=w1581, "Item Symbols"=w1583) -> ()  [unwired: 2 in, 2 out]
                n1320 = property on="Diff Test Items" class="LstBox (严格)"("Value"=w1572, "Top Row"=w1572) -> ()  [unwired: 2 in, 2 out]
                n1321 = property on="Single Test Items" class="LstBox (严格)"("Value"=w1572, "Top Row"=w1572) -> ()  [unwired: 2 in, 2 out]
                n1322 = property on="TDR Test Items" class="LstBox (严格)"("Value"=w1572, "Top Row"=w1572) -> ()  [unwired: 2 in, 2 out]
                n1323 = property on="NEXT Pair Name" class="LstBox (严格)"("Value"=w1572, "Top Row"=w1572) -> ()  [unwired: 2 in, 2 out]
                n1324 = property on="FEXT Pair Name" class="LstBox (严格)"("Value"=w1572, "Top Row"=w1572) -> ()  [unwired: 2 in, 2 out]
                n1325 = property on="S-para Pair Name" class="LstBox (严格)"("Value"=w1572, "Top Row"=w1572) -> ()  [unwired: 2 in, 2 out]
              }
            }
          }
          event "Default  fre": Value Change {
            n1326 = event-data() -> ()  [unwired: 1 in, 5 out]
            n1327 = case shown="\"Clear\"" "Default  fre" {
              frame "Default", Default {
                n1328 = local write "fre-save"(string[] ["2500", "4500", "5000", "5156.25", "6000", "9000", "10000", "12890", "19000", "20000"]) -> ()
              }
              frame "Clear" {
                n1329 = local write "fre-save"(string[] [] ("fre-save")) -> ()
              }
            }
          }
          event "Default": Value Change {
            n1330 = event-data() -> ()  [unwired: 1 in, 5 out]
            n1331 = case shown="真" "Default" {
              frame False {
              }
              frame True {
                n1332 = property on="Postion for \"PN&Tester&Date\" etc Fields" class="Tbl (严格)"("Value"=string[][] [["Applicant", "0", "2", "1"], ["Part Name", "0", "3", "1"], ["Part Number", "0", "4", "1"], ["Report No", "0", "2", "12"], ["Sample No", "0", "4", "12"], ["Prepared By", "0", "63", "0"], ["Approved By", "0", "63", "6"], ["Date", "0", "63", "2"], ["Thru Result", "0", "13", "5"], ["NEXT Result", "0", "45", "4"], ["FEXT Result", "0", "45", "5"]] ("Postion for \"PN&Tester&Date\" etc Fields"), "Active Cell"=T4 {"Row"=0, "Column"=0} ("编辑位置")) -> ()  [unwired: 2 in, 2 out]
              }
            }
          }
        }
      }
    }
  }
